vi "enumerateStaticDependencies.vi"(8 "error in (no error)":errorcluster, 11 "SMO.E":refnum<class "SMO.E.lvclass">) -> (0 "error out":errorcluster, 2 "Static Dependencies":refnum<class "Dependency.lvclass">[](array[class]), 3 "SMO.E out":refnum<class "SMO.E.lvclass">)   [LabVIEW 2013, in "SMO.E.lvclass"]
uses:
  SMO.E.lvclass
  src/Dependency/Dependency.lvclass
  SMO.B/SMO.B.lvclass
  src/SMO/SMO.lvclass
panel:
  # "For instructions on how to use the JKI State Machine Objects, examples and video tutorials, visit:\nhttp://jki.net/state-machine-objects/\n\nJKI State Machine Objects™\nhttp://jki.net/state-machine-objects/\nCopyright (C) 2005-2015, JKI <info@jki.net>\nALL RIGHTS RESERVED"
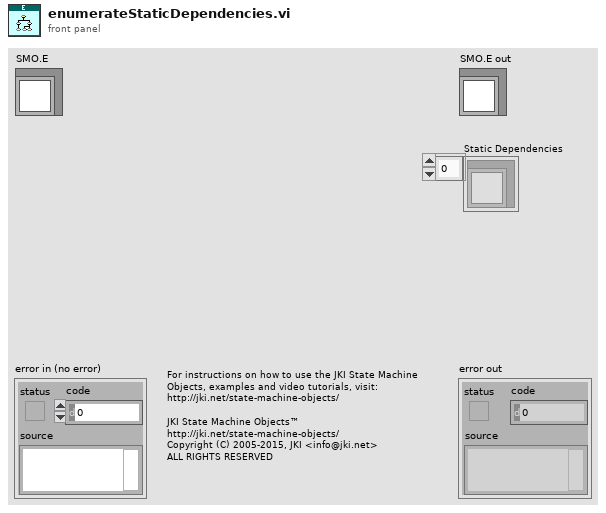
[diagram p1: front panel]
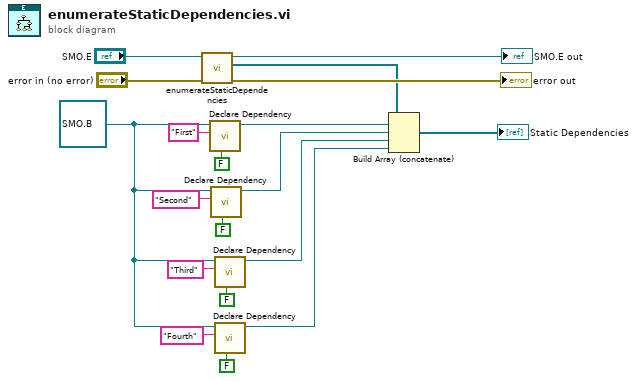
[diagram p0: block diagram]
diagram:
  w4 = refnum<class "SMO.B.lvclass"> refnum ("SMO.B.lvclass")
  n1 = call-parent "enumerateStaticDependencies.vi"("error in (no error)"="error in (no error)", "SMO"="SMO.E") -> ("error out"=→"error out":errorcluster, "Static Dependencies"=w12:refnum<class "Dependency.lvclass">[], "SMO out"=→"SMO.E out":refnum<class "SMO.E.lvclass">)  [unwired: 7 in]
  n2 = call "Declare Dependency.vi"("Shared Resource (F)"=FALSE, "Name"="First", "Type"=w4) -> ("Dependency out"=w13:refnum<class "Dependency.lvclass">)  [unwired: 7 in, 1 out]
  n3 = call "Declare Dependency.vi"("Shared Resource (F)"=FALSE, "Name"="Second", "Type"=w4) -> ("Dependency out"=w3:refnum<class "Dependency.lvclass">)  [unwired: 7 in, 1 out]
  n4 = call "Declare Dependency.vi"("Shared Resource (F)"=FALSE, "Name"="Third", "Type"=w4) -> ("Dependency out"=w2:refnum<class "Dependency.lvclass">)  [unwired: 7 in, 1 out]
  n5 = call "Declare Dependency.vi"("Shared Resource (F)"=FALSE, "Name"="Fourth", "Type"=w4) -> ("Dependency out"=w1:refnum<class "Dependency.lvclass">)  [unwired: 7 in, 1 out]
  n6 = Build Array (concatenate)(w12, w13, w3, w2, w1) -> (→"Static Dependencies":refnum<class "Dependency.lvclass">[])
